vi "_Insert a New Node.vi"(6 "Data":string="False", 7 "Tag Name":string="ESI2", 8 "error in (no error)":errorcluster, 9 "Reference Child":refnum<k20>, 10 "Experiment Node":refnum<k20>, 11 "DOM Document":refnum<k20>) -> (0 "error out":errorcluster, 1 "Reference Child out":refnum<k20>, 2 "Experiment Node out":refnum<k20>, 3 "DOM Document out":refnum<k20>)   [LabVIEW 2012]
uses:
  <vilib>/xml/Close Reference(Node).vi
  <resource>/objmgr/DOMUserDefRef.rc
  <vilib>/xml/NI_XML.lvlib
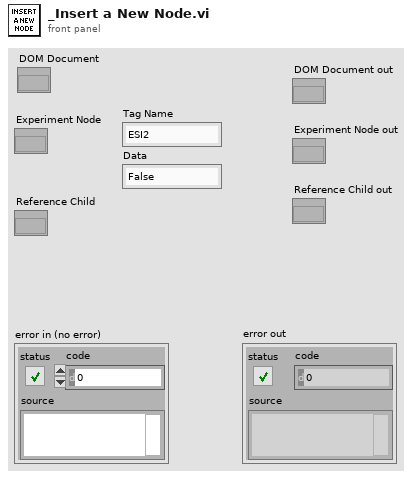
[diagram p1: front panel]
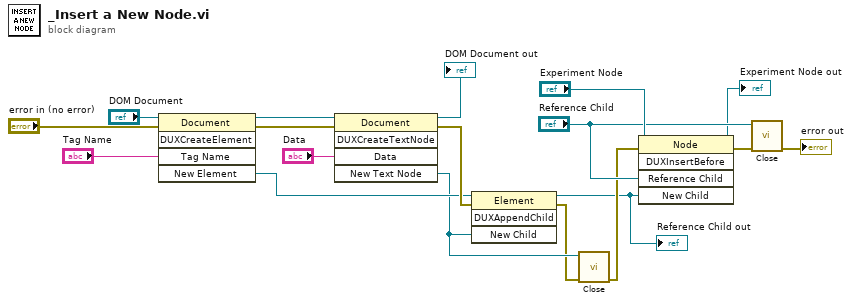
[diagram p0: block diagram]
diagram:
  n1 = invoke class="Document" method="DUXCreateElement"(reference="DOM Document", error in="error in (no error)", "Tag Name"="Tag Name") -> (reference out=w16:refnum<k20>, error out=w15:errorcluster, "New Element"=w12:refnum<k20>)  [unwired: 2 in, 2 out]
  n2 = invoke class="Document" method="DUXCreateTextNode"(reference=w16, error in=w15, "Data"="Data") -> (reference out=→"DOM Document out":refnum<k20>, error out=w13:errorcluster, "New Text Node"=w8:refnum<k20>)  [unwired: 2 in, 2 out]
  n3 = invoke class="Element" method="DUXAppendChild"(reference=w12, error in=w13, "New Child"=w8) -> (reference out=w2:refnum<k20>, error out=w7:errorcluster)  [unwired: 1 in, 2 out]
  "Reference Child out" <- w2
  n4 = call-poly <vilib>:"Close.vi"("error in (no error)"=w7, "node"=w8) -> ("error out"=w6:errorcluster)  [unwired: 7 out]
  n5 = invoke class="Node" method="DUXInsertBefore"(reference="Experiment Node", error in=w6, "Reference Child"="Reference Child", "New Child"=w2) -> (reference out=→"Experiment Node out":refnum<k20>, error out=w5:errorcluster)  [unwired: 1 in, 3 out]
  n6 = call-poly <vilib>:"Close.vi"("error in (no error)"=w5, "node"="Reference Child") -> ("error out"=→"error out":errorcluster)  [unwired: 7 out]
